vi "Memory.Pointer.Offset to Address.vi"   [LabVIEW 2016, in "LabVIEW Memory Manager.lvlib" / "Memory.Pointer.Void.lvclass"]
uses:
  Memory.Pointer.Void.lvclass
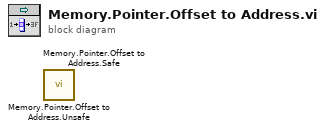
[diagram p0: block diagram]
diagram:
  n1 = call "Memory.Pointer.Offset to Address.Unsafe.vi"() -> ()  [unwired: 9 in, 3 out]
  n2 = call "Memory.Pointer.Offset to Address.Safe.vi"() -> ()  [unwired: 9 in, 3 out]
